vi "Model - Init.vi"(8 "error in (no error)":errorcluster) -> (0 "error out":errorcluster, 3 "View Model":T1)   [LabVIEW 2013]
doc: "Initializes the View Model."
uses:
  Controls/View Model.ctl
  Error/Controls/Error Model.ctl
  Error/Controls/Error Types.ctl
  Controls/Shared Model.ctl
  Elevator Controller/Controls/Elevator Model.ctl
  Elevator Controller/Controls/Controller Overhead.ctl
  Elevator Controller/Controls/Elevator States.ctl
  Elevator Controller/Controls/Elevator Location.ctl
  Elevator Controller/Controls/Elevator Command Event.ctl
  Elevator Controller/Controls/Elevator Commands.ctl
  Configuration/Controls/Configuration Model.ctl
  Configuration/Controls/Configuration Data.ctl
  Error/Controls/Error Event Data.ctl
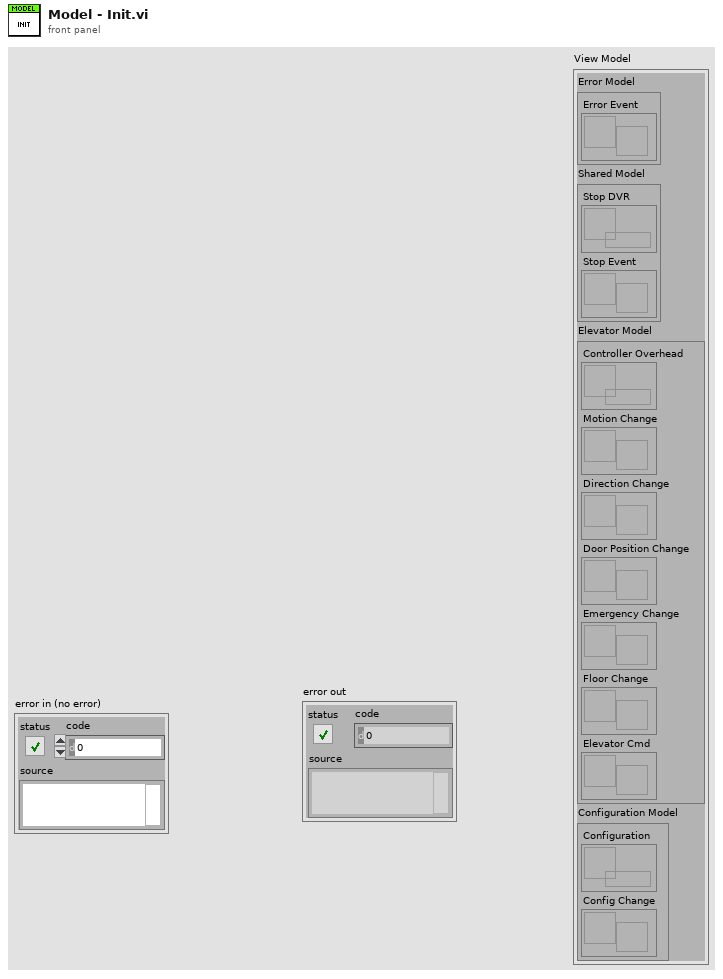
[diagram p1: front panel]
types:
  T1 = typedef "View Model.ctl" = cluster{"Error Model":T2, "Shared Model":T3, "Elevator Model":T4, "Configuration Model":T5}
  T2 = typedef "Error Model.ctl" = cluster{"Error Event":refnum<user-event>}
  T3 = typedef "Shared Model.ctl" = cluster{"Stop DVR":refnum<data-value>, "Stop Event":refnum<user-event>}
  T4 = typedef "Elevator Model.ctl" = cluster{"Controller Overhead":refnum<data-value>, "Motion Change":refnum<user-event>, "Direction Change":refnum<user-event>, "Door Position Change":refnum<user-event>, "Emergency Change":refnum<user-event>, "Floor Change":refnum<user-event>, "Elevator Cmd":refnum<user-event>}
  T5 = typedef "Configuration Model.ctl" = cluster{"Configuration":refnum<data-value>, "Config Change":refnum<user-event>}
  T6 = typedef "Elevator Command Event.ctl" = cluster{"Elevator Commands":T7, "Variant":variant}
  T7 = typedef "Elevator Commands.ctl" = enum16{"Go Up", "Go Down", "Go To Floor", "Emergency", "Open Doors", "Close Doors"}
  T8 = typedef "Elevator Location.ctl" = enum16{"1st Floor", "2nd Floor", "3rd Floor", "4th Floor"}
  T9 = typedef "Controller Overhead.ctl" = cluster{"In Motion?":bool, "Direction":bool, "Door Movement":bool, "Elevator State":T10, "Next Elevator State":T10, "Timer":dbl, "Elapsed Time":dbl, "Door Position":bool}
  T10 = typedef "Elevator States.ctl" = enum16{"Initial State", "Open Doors", "Close Doors", "Start Move", "Move", "Finish Move", "Emergency", "Analysis"}
  T11 = typedef "Error Event Data.ctl" = cluster{"Error Type":T12, "error in (no error)":errorcluster}
  T12 = typedef "Error Types.ctl" = enum16{"Console Error", "Process Step Error", "Sensor Interface IO Error"}
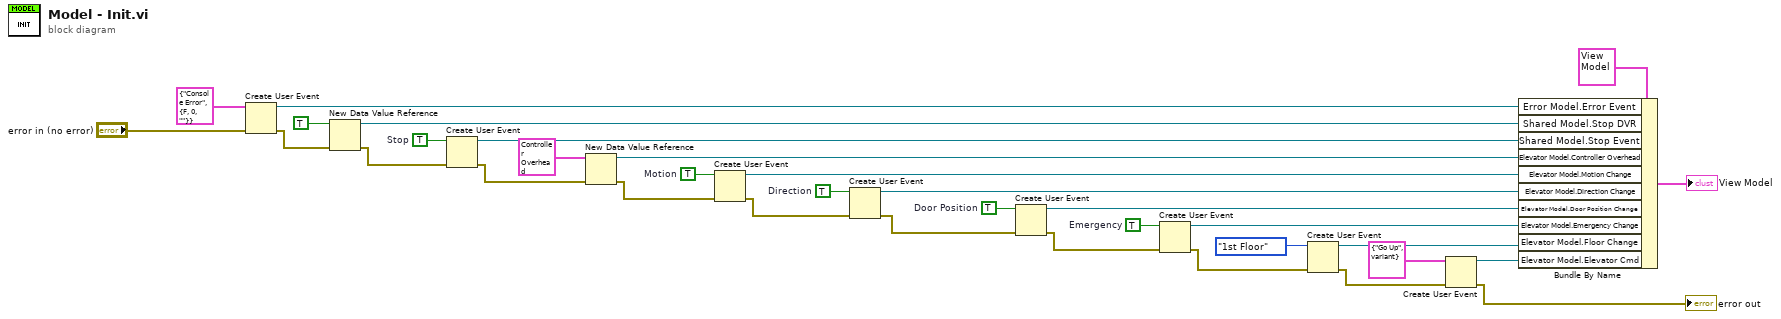
[diagram p0: block diagram]
diagram:
  w11 = TRUE  # Emergency
  w14 = TRUE  # Door Position
  w17 = TRUE  # Direction
  w19 = TRUE  # Motion
  w26 = TRUE  # Stop
  n1 = Create User Event(user event datatype=T11 {"Error Type"=enum."Console Error", "error in (no error)"={"status"=FALSE, "code"=0, "source"=""}} ("Error Event Data"), error in="error in (no error)") -> (user event=w31:refnum<user-event>, error out=w27:errorcluster)
  n2 = New Data Value Reference(data value=TRUE, error in=w27) -> (data value reference=w28:refnum<data-value>, error out=w24:errorcluster)
  n3 = Create User Event(user event datatype=w26, error in=w24) -> (user event=w25:refnum<user-event>, error out=w22:errorcluster)
  n4 = New Data Value Reference(data value=T9 {"In Motion?"=FALSE, "Direction"=FALSE, "Door Movement"=FALSE, "Elevator State"=enum."Initial State", "Next Elevator State"=enum."Initial State", "Timer"=0.0, "Elapsed Time"=0.0, "Door Position"=FALSE} ("Controller Overhead"), error in=w22) -> (data value reference=w21:refnum<data-value>, error out=w18:errorcluster)
  n5 = Create User Event(user event datatype=w19, error in=w18) -> (user event=w20:refnum<user-event>, error out=w16:errorcluster)
  n6 = Create User Event(user event datatype=w17, error in=w16) -> (user event=w15:refnum<user-event>, error out=w13:errorcluster)
  n7 = Create User Event(user event datatype=w14, error in=w13) -> (user event=w12:refnum<user-event>, error out=w9:errorcluster)
  n8 = Create User Event(user event datatype=w11, error in=w9) -> (user event=w10:refnum<user-event>, error out=w8:errorcluster)
  n9 = Create User Event(user event datatype=Elevator_Location."1st Floor" ("Elevator Location"), error in=w8) -> (user event=w7:refnum<user-event>, error out=w2:errorcluster)
  n10 = Create User Event(user event datatype=T6 {"Elevator Commands"=enum."Go Up", "Variant"=variant} ("Elevator Cmd Event"), error in=w2) -> (user event=w4:refnum<user-event>, error out=→"error out":errorcluster)
  n11 = Bundle By Name(cluster=T1 {"Error Model"={"Error Event"=refnum}, "Shared Model"={"Stop DVR"=refnum, "Stop Event"=refnum}, "Elevator Model"={"Controller Overhead"=refnum, "Motion Change"=refnum, "Direction Change"=refnum, "Door Position Change"=refnum, "Emergency Change"=refnum, "Floor Change"=refnum, "Elevator Cmd"=refnum}, "Configuration Model"={"Configuration"=refnum, "Config Change"=refnum}} ("View Model"), "Error Model.Error Event"=w31, "Shared Model.Stop DVR"=w28, "Shared Model.Stop Event"=w25, "Elevator Model.Controller Overhead"=w21, "Elevator Model.Motion Change"=w20, "Elevator Model.Direction Change"=w15, "Elevator Model.Door Position Change"=w12, "Elevator Model.Emergency Change"=w10, "Elevator Model.Floor Change"=w7, "Elevator Model.Elevator Cmd"=w4) -> (→"View Model":T1)
